vi "DHE_ReadModes.vi"(8 "error in (no error)":errorcluster, 9 "read mode":string, 10 "configuration file path":path, 11 "fd":i32) -> (0 "error out":errorcluster, 2 "error_code":i32, 3 "fd out":i32)   [LabVIEW 2016]
uses:
  <vilib>/Utility/config.llb/Read Key (String).vi
  <vilib>/Utility/config.llb/NI_LVConfig.lvlib
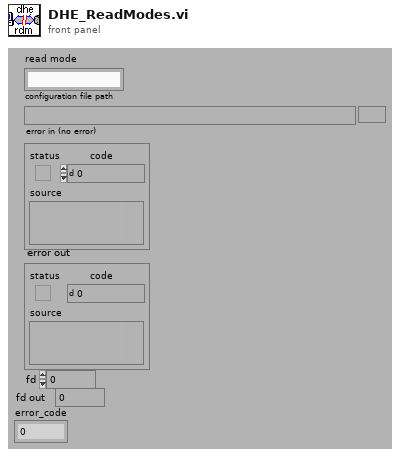
[diagram p1: front panel]
types:
  T1 = typedef "NI_LVConfig.lvlib/Config Data RefNum.ctl" = refnum<k1>
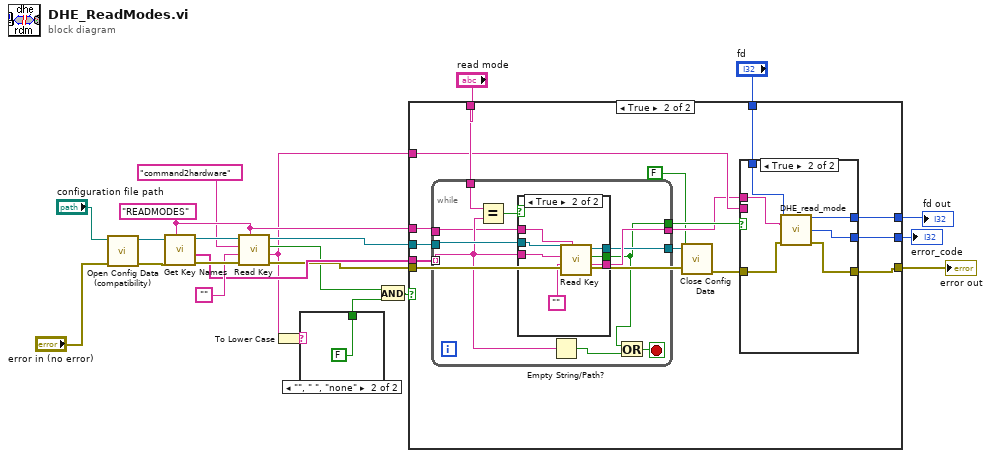
[diagram p0: block diagram]
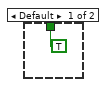
[diagram p2: hidden frame]
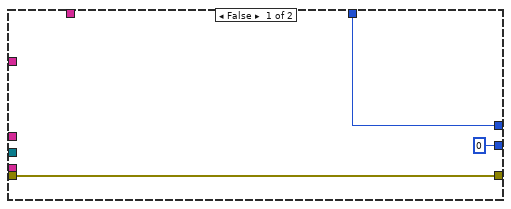
[diagram p3: hidden frame]
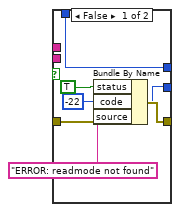
[diagram p4: hidden frame]
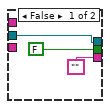
[diagram p5: hidden frame]
diagram:
  w13 = "READMODES" ("section")
  n1 = call <vilib>:"Open Config Data (compatibility).vi"("error in (no error)"="error in (no error)", "configuration file path"="configuration file path") -> ("error out"=w21:errorcluster, "refnum"=w20:T1)  [unwired: 7 in, 1 out]
  n2 = call <vilib>:"Get Key Names.vi"("section"=w13, "error in (no error)"=w21, "refnum"=w20) -> ("error out"=w17:errorcluster, "key names"=w14:string[], "refnum out"=w18:T1)  [unwired: 6 out]
  n3 = call-poly <vilib>:"Read Key.vi"("section"=w13, "error in (no error)"=w17, "default value"="", "key"="command2hardware", "refnum"=w18) -> ("error out"=w11:errorcluster, "value"=w4:string, "found?"=w5:bool, "refnum out"=w15:T1)  [unwired: 1 in, 2 out]
  n4 = To Lower Case(string=w4) -> (all lower case string=w3:string)
  n5 = case shown="\"\", \" \", \"none\"" w3 {
    tunnel: [TRUE FALSE] -> w2
    frame Default {
    }
    frame "", " ", "none" {
    }
  }
  n6 = And(x=w5, y=w2) -> (x .and. y?=w6:bool)
  n7 = case shown="True" w6 {
    tunnel: "read mode" -> [_ w42]
    tunnel: w15 -> [_ w41]
    tunnel: w14 -> [_ w40]
    tunnel: w13 -> [_ w39]
    tunnel: w11 -> [w27 w37]
    tunnel: [w27 w34] -> w10
    tunnel: "fd" -> [w26 w33]
    tunnel: [w26 w32] -> w8
    tunnel: w4 -> [_ w31]
    tunnel: [0 w29] -> w1
    frame False {
    }
    frame True {
      n8 = while {
        tunnel: w40 -> [w60] mode=indexing
        tunnel: w41 -> [w64]
        tunnel: w39 -> [w57]
        tunnel: w42 -> [w63]
        tunnel: [w61] -> w30
        tunnel: [w58] -> w38
        tunnel: [w55] -> w36
        stop <- w56 stop-if-true
        n9 = Equal?(x=w63, y=w60) -> (x = y?=w62:bool)
        n10 = case shown="True" w62 {
          tunnel: w64 -> [w66 w74]
          tunnel: w57 -> [_ w72]
          tunnel: w60 -> [_ w71]
          tunnel: ["" w70] -> w61
          tunnel: [w66 w69] -> w58
          tunnel: [FALSE ("found?") w68] -> w55
          frame False {
          }
          frame True {
            n11 = call-poly <vilib>:"Read Key.vi"("section"=w72, "default value"="", "key"=w71, "refnum"=w74) -> ("value"=w70:string, "found?"=w68:bool, "refnum out"=w69:T1)  [unwired: 2 in, 3 out]
          }
        }
        n12 = Empty String/Path?(string/path=w60) -> (empty?=w59:bool)
        n13 = Or(x=w55, y=w59) -> (x .or. y?=w56:bool)
      }
      n14 = call <vilib>:"Close Config Data.vi"("error in (no error)"=w37, "write file if changed (T)"=FALSE ("write configuration file? (T)"), "refnum"=w38) -> ("error out"=w35:errorcluster)  [unwired: 8 out]
      n15 = case shown="True" w36 {
        tunnel: w35 -> [w46 w52]
        tunnel: [w44 w51] -> w34
        tunnel: w33 -> [w48 w54]
        tunnel: [w48 w53] -> w32
        tunnel: w31 -> [_ _]
        tunnel: w30 -> [_ w49]
        tunnel: [w43 w50] -> w29
        frame False {
          w43 = -22 ("code")
          n16 = Bundle By Name(cluster=w46, "status"=TRUE, "code"=w43, "source"="ERROR: readmode not found") -> (w44:errorcluster)
        }
        frame True {
          n17 = call "DHE_read_mode.vi"("fd"=w54, "mode"=w49, "error in (no error)"=w52) -> ("fd out"=w53:i32, "return value"=w50:i32, "error out"=w51:errorcluster)  [unwired: 10 out]
        }
      }
    }
  }
  "error out" <- w10
  "fd out" <- w8
  "error_code" <- w1
